vi "Describe Call Comparison.vi"(10 "VI Call 2":refnum<class "VI Call.lvclass">, 11 "VI Call in":refnum<class "VI Call.lvclass">) -> (3 "delimited string":string)   [LabVIEW 2020, in "Identical Inputs Comparator.lvclass"]
uses:
  Identical Inputs Comparator.lvclass
  Core/VI Call/VI Call.lvclass
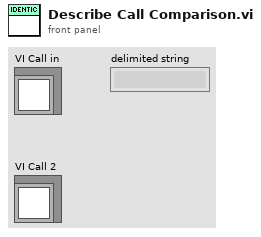
[diagram p1: front panel]
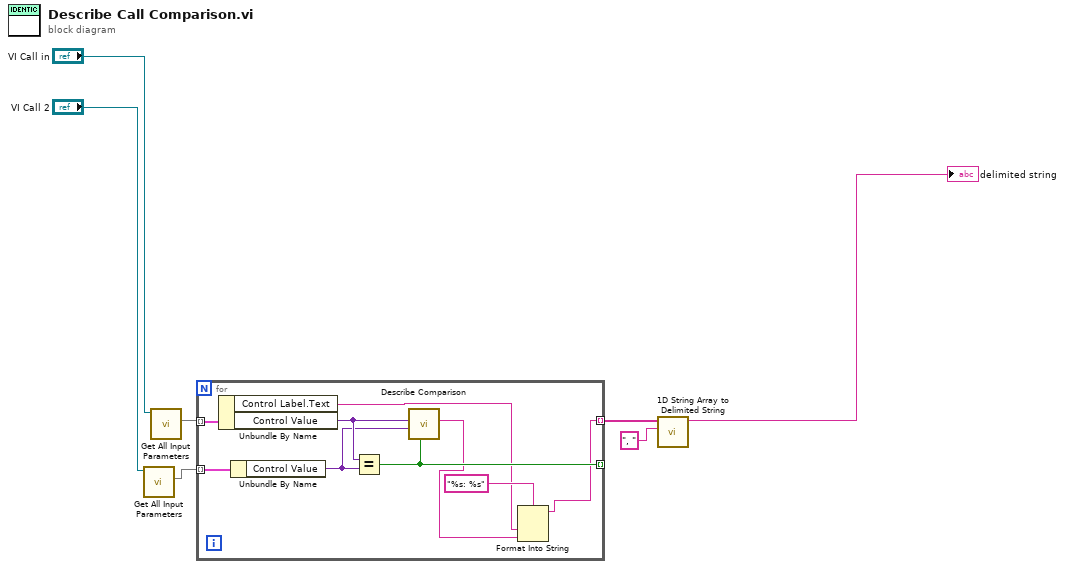
[diagram p0: block diagram]
diagram:
  n1 = call-dynamic "Get All Input Parameters.vi"("VI Call in"="VI Call 2") -> ("Input Parameters"=w6:map{string, variant})  [unwired: 9 in, 1 out]
  n2 = call-dynamic "Get All Input Parameters.vi"("VI Call in"="VI Call in") -> ("Input Parameters"=w4:map{string, variant})  [unwired: 9 in, 1 out]
  n3 = for {
    tunnel: w4 -> [w16] mode=indexing
    tunnel: w6 -> [w15] mode=indexing
    tunnel: [w12] -> _ mode=indexing
    tunnel: [w8] -> w1 mode=indexing
    n4 = Unbundle By Name(w16) -> ("Control Label.Text"=w9:string, "Control Value"=w14:variant)
    n5 = Unbundle By Name(w15) -> ("Control Value"=w13:variant)
    n6 = Equal?(x=w14, y=w13) -> (x = y?=w12:bool)
    n7 = call "Describe Comparison.vi"("Equal?"=w12, "Control Value 2"=w13, "Control Value 1"=w14) -> ("Description"=w10:string)  [unwired: 7 in, 1 out]
    n8 = Format Into String(format string="%s: %s", w9, w10) -> (resulting string=w8:string)  [unwired: 2 in, 1 out]
  }
  n9 = call <vilib>:"1D String Array to Delimited String.vi"("delimiter"=", ", "string array"=w1) -> ("delimited string"=→"delimited string":string)  [unwired: 9 in]
